vi "LDA_analogue_start_time_sync_PN.vi"(0 "Burst detect HW delay (s)":dbl=0.008, 4 "Correlation peak fit method":enum32{"Max", "Quadratic", "Gaussian"}(ring)=enum."Quadratic", 5 "Pulse high threshold (Volts)":dbl=2.5, 6 "Analogue dt (s)":dbl, 7 "Analogue LDA burst pulse array":dbl[](array[numeric]), 8 "LDA arrival Times":dbl[](array[numeric])) -> (1 "valid bursts checksum status":bool=TRUE, 2 "Absolute LDA times (s)":dbl[](array[numeric]), 3 "LDA start time rel. to Analogue (s)":dbl)   [LabVIEW 2011]
uses:
  <vilib>/Analysis/1siggen.llb/Ramp Pattern by Samples.vi
  <vilib>/Analysis/2dsp.llb/1D Cross Correlation (DBL).vi
  <vilib>/Analysis/polynomials.llb/Polynomial Roots (DBL).vi
  <vilib>/Analysis/polynomials.llb/nth Derivative of Polynomial (DBL).vi
  <vilib>/Analysis/NI_AALPro.lvlib
  <vilib>/Analysis/NI_AALBase.lvlib
panel:
  out "Xcorr LDA timings":cluster{"Ramp Pattern":dbl[], dbl[]}[](graph)
  in  "Pts. either side of peak to use in fit":i32=3
  out "Analogue LDA burst pulse array":cluster{"index (row)":dbl, dbl, "Vout":dbl[]}(graph)
  out "Thresholded LDA burst times (valid only)":cluster{"index (row)":dbl, dbl, "Vout":dbl[]}(graph)
  out "Thresholded LDA arr time checksum":i32
  out "Thresholded LDA burst times (valid + invalid)":cluster{"index (row)":dbl, dbl, "Vout":dbl[]}(graph)
  out "LDA counted pulses (valid + invalid)":i32
  out "LDA arr_t length":i32
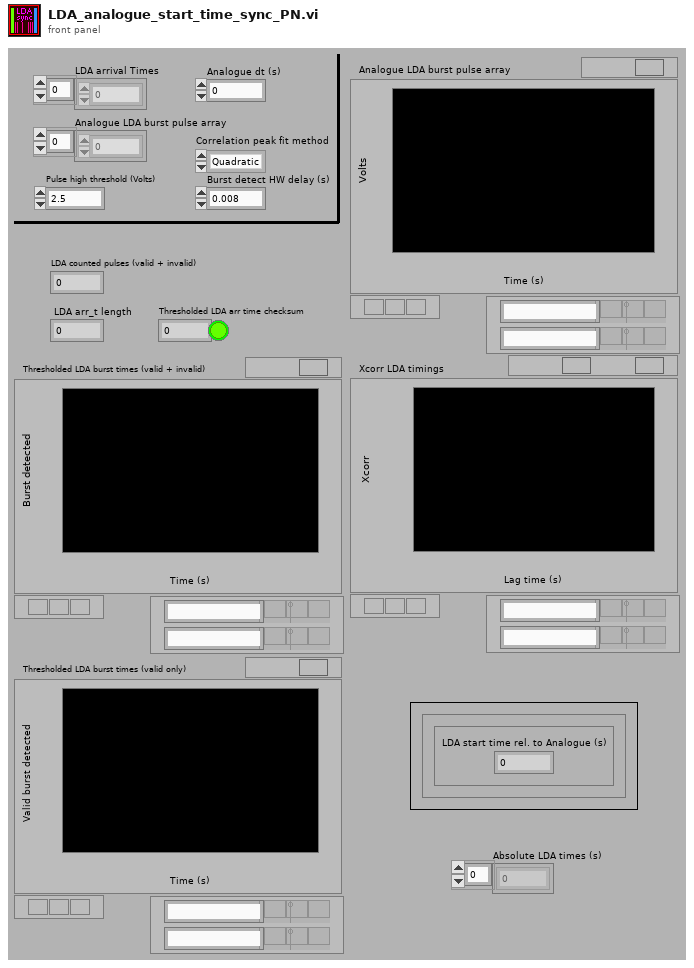
[diagram p1: front panel]
types:
  T1 = cluster{"index (row)":dbl, "Analogue dt (s)":dbl, "Vout":dbl[]}
  T2 = cluster{"index (row)":dbl, "Analogue dt (s)":dbl, "Analogue LDA burst pulse array":dbl[]}
  T3 = cluster{"Ramp Pattern":dbl[], "Best Gaussian Fit":dbl[]}[]
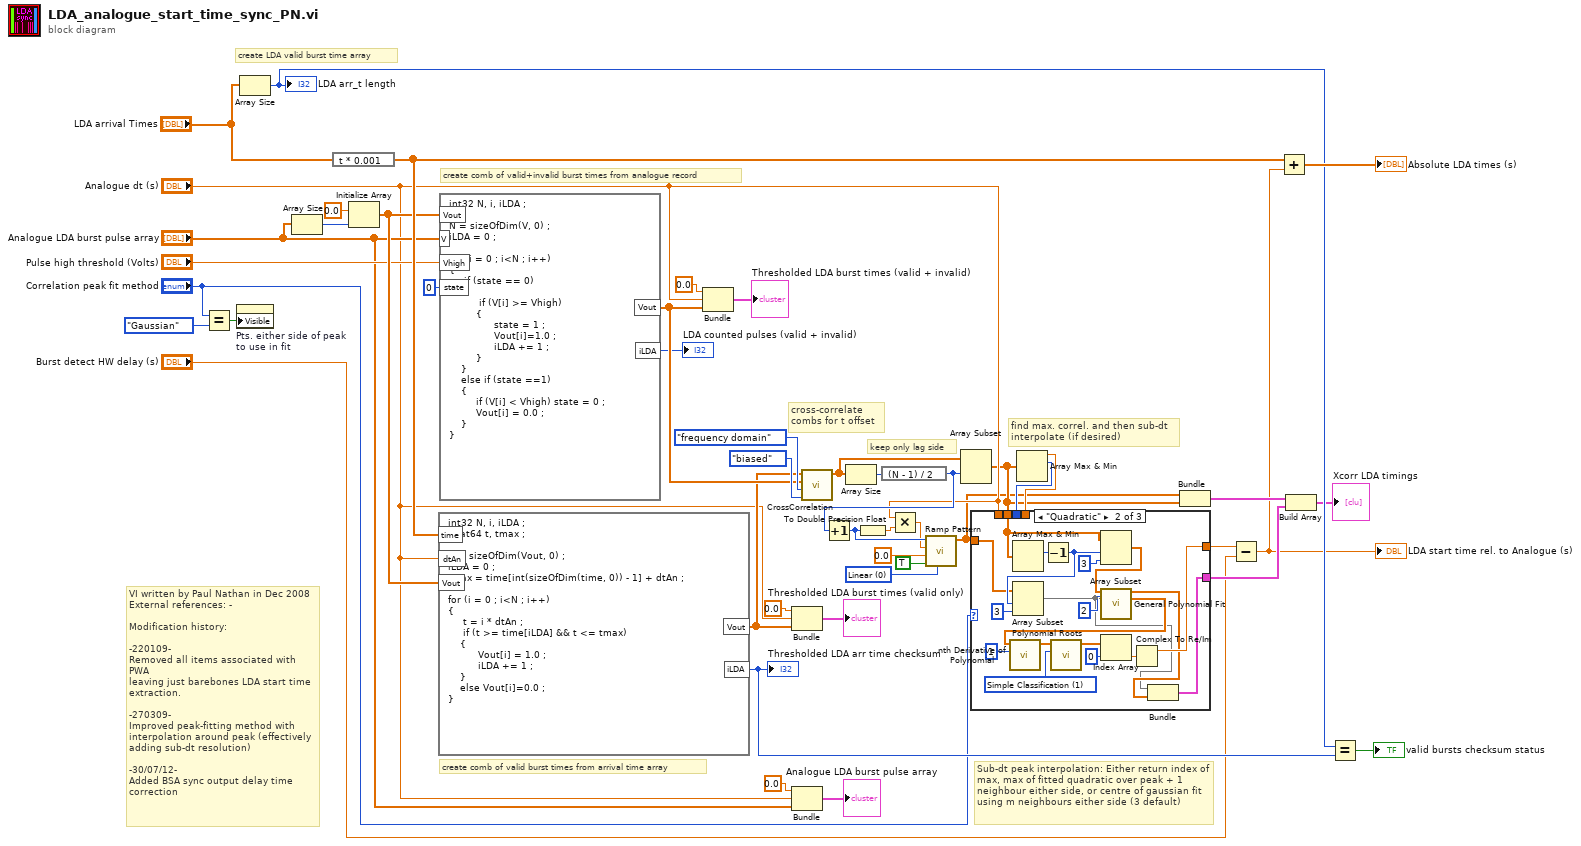
[diagram p0: block diagram]
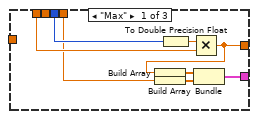
[diagram p2: hidden frame]
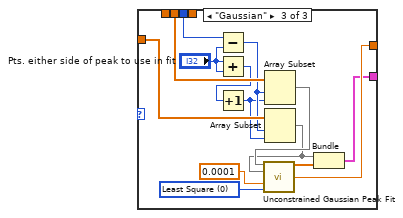
[diagram p3: hidden frame]
diagram:
  w13 = u16 0 items=["Linear", "Logarithmic"] ("type")
  # "find max. correl. and then sub-dt interpolate (if desired)"
  # "Sub-dt peak interpolation: Either return index of max, max of fitted quadratic over peak + 1 neighbour either side, or centre of gaussian fit using m neighbours either side (3 default)"
  # "create LDA valid burst time array"
  # "keep only lag side"
  # "cross-correlate combs for t offset"
  # "VI written by Paul Nathan in Dec 2008\nExternal references: -\n\nModification history:\n\n-220109-\nRemoved all items associated with PWA\nleaving just barebones LDA start time\nextraction.\n\n-270309-\nImproved peak-fitting method with interpolation around peak (effectively adding sub-dt resolution)\n\n-30/07/12-\nAdded BSA sync output delay time correction"
  # "create comb of valid+invalid burst times from analogue record"
  # "create comb of valid burst times from arrival time array"
  n1 = Equal?(x="Correlation peak fit method", y=enum32{"Max", "Quadratic", "Gaussian"}."Gaussian") -> (x = y?=w6:bool)
  n2 = property on="Pts. either side of peak to use in fit" class="DigNum (strict)"("Visible"=w6) -> ()  [unwired: 2 in, 2 out]
  n3 = Array Size(array="LDA arrival Times") -> (size(s)=w28:i32)
  "LDA arr_t length" <- w28
  n4 = Array Size(array="Analogue LDA burst pulse array") -> (size(s)=w33:i32)
  n5 = expression code="t * 0.001"("LDA arrival Times") -> (w34:dbl[])
  n6 = Initialize Array(0.0 ("element"), w33) -> (w32:dbl[])
  n7 = formula code="int32 N, i, iLDA ;\nfloat64 t, tmax ;\n\nN = sizeOfDim(Vout, 0) ;\niLDA = 0 ;\ntmax = time[int(sizeOfDim(time, 0)) - 1] + dtAn ;\n\nfor (i = 0 ; i<N ; i++)\n{\n     t = i * dtAn ;\n     if (t >= time[iLDA] && t <= tmax) \n    {\n          Vout[i] = 1.0 ;\n          iLDA += 1 ;\n    }\n    else Vout[i]=0.0 ;\n}"("dtAn"="Analogue dt (s)", "time"=w34, "Vout"=w32) -> ("Vout"=w37:dbl[], "iLDA"=w31:i32)
  "Thresholded LDA arr time checksum" <- w31
  n8 = formula code="int32 N, i, iLDA ;\n\nN = sizeOfDim(V, 0) ;\niLDA = 0 ;\n\nfor (i = 0 ; i<N ; i++)\n{\n     if (state == 0) \n    {\n          if (V[i] >= Vhigh)\n         {\n               state = 1 ;\n               Vout[i]=1.0 ;\n               iLDA += 1 ;\n         }\n    }\n    else if (state ==1)\n    {\n         if (V[i] < Vhigh) state = 0 ;\n         Vout[i] = 0.0 ;\n    }\n}"("V"="Analogue LDA burst pulse array", "Vhigh"="Pulse high threshold (Volts)", "state"=u8 0 ("input variable"), "Vout"=w32) -> ("Vout"=w38:dbl[], "iLDA"=→"LDA counted pulses (valid + invalid)":i32)
  n9 = Bundle("index (row)"=0.0, "Analogue dt (s)"="Analogue dt (s)", "Vout"=w38) -> (→"Thresholded LDA burst times (valid + invalid)":T1)  [unwired: 1 out]
  n10 = Bundle("index (row)"=0.0, "Analogue dt (s)"="Analogue dt (s)", "Vout"=w37) -> (→"Thresholded LDA burst times (valid only)":T1)  [unwired: 1 out]
  n11 = Bundle("index (row)"=0.0, "Analogue dt (s)"="Analogue dt (s)", "Analogue LDA burst pulse array"="Analogue LDA burst pulse array") -> (→"Analogue LDA burst pulse array":T2)  [unwired: 1 out]
  n12 = call-poly <vilib>:"CrossCorrelation.vi"("normalization"=enum32{"none", "unbiased", "biased"}."biased", "algorithm"=enum32{"direct", "frequency domain"}."frequency domain", "Y"=w38, "X"=w37) -> ("Rxy"=w35:dbl[])  [unwired: 7 out]
  n13 = Array Size(array=w35) -> (size(s)=w36:i32)
  n14 = expression code="(N - 1) / 2"(w36) -> (w15:i32)
  n15 = Increment(x=w15) -> (x+1=w22:i32)
  n16 = To Double Precision Float(number=w22) -> (double precision float=w20:dbl)
  n17 = Multiply(x="Analogue dt (s)", y=w20) -> (x*y=w21:dbl)
  n18 = call-poly <vilib>:"Ramp Pattern.vi"("type"=w13, "exclude end?"=TRUE, "start"=0.0, "end"=w21, "samples"=w22) -> ("Ramp Pattern"=w9:dbl[])  [unwired: 5 in, 1 out]
  n19 = Array Subset(array=w35, index=w15) -> (w10:dbl[])  [unwired: 1 in]
  n20 = Array Max & Min(array=w10) -> (max value=w11:dbl, max index (indices)=w12:i32)  [unwired: 2 out]
  n21 = case shown="\"Quadratic\"" "Correlation peak fit method" {
    tunnel: w10 -> [_ w62 w84]
    tunnel: [w47 w63 w86] -> w3
    tunnel: "Analogue dt (s)" -> [w54 _ _]
    tunnel: [w51 w60 w76] -> w8
    tunnel: w9 -> [_ w56 w81]
    tunnel: w12 -> [w52 _ w83]
    tunnel: w11 -> [w48 _ _]
    frame "Max" {
      n22 = Build Array(w48) -> (w50:dbl[])
      n23 = To Double Precision Float(number=w52) -> (double precision float=w53:dbl)
      n24 = Multiply(x=w53, y=w54) -> (x*y=w47:dbl)
      n25 = Build Array(w47) -> (w49:dbl[])
      n26 = Bundle(w49, w50) -> (w51:cluster{dbl[], dbl[]})  [unwired: 1 out]
    }
    frame "Quadratic" {
      w67 = u16 1 items=["General", "Simple Classification", "Refinement", "Advanced Refinement"] ("option")
      n27 = Array Max & Min(array=w62) -> (max index (indices)=w72:i32)  [unwired: 3 out]
      n28 = Decrement(x=w72) -> (x-1=w57:i32)
      n29 = Array Subset(array=w56, index=w57, length=3) -> (w55:dbl[])
      n30 = Array Subset(array=w62, index=w57, length=3) -> (w71:dbl[])
      n31 = call <vilib>:"General Polynomial Fit.vi"("Y"=w71, "polynomial order"=2, "X"=w55) -> ("Best Polynomial Fit"=w59:dbl[], "Polynomial Coefficients"=w61:dbl[])  [unwired: 9 in, 2 out]
      n32 = call-poly <vilib>:"nth Derivative of Polynomial.vi"("order"=1, "P(x)"=w61) -> ("Nth Derivative of P(x)"=w68:dbl[])  [unwired: 9 out]
      n33 = call-poly <vilib>:"Polynomial Roots.vi"("option"=w67, "P(x)"=w68) -> ("Roots"=w66:cdb[])  [unwired: 9 out]
      n34 = Index Array(array=w66, index=0) -> (element=w64:cdb)
      n35 = Complex To Re/Im(x + iy=w64) -> (x=w63:dbl)  [unwired: 1 out]
      n36 = Bundle(w55, "Best Polynomial Fit"=w59) -> (w60:cluster{dbl[], "Best Polynomial Fit":dbl[]})  [unwired: 1 out]
    }
    frame "Gaussian" {
      w85 = u16 0 items=["Least Square", "Least Absolute Residual", "Bisquare"] ("method")
      n37 = Subtract(x=w83, y="Pts. either side of peak to use in fit") -> (x-y=w80:i32)
      n38 = Add(x="Pts. either side of peak to use in fit", y="Pts. either side of peak to use in fit") -> (x+y=w74:i32)
      n39 = Increment(x=w74) -> (x+1=w75:i32)
      n40 = Array Subset(array=w84, index=w80, length=w75) -> (w79:dbl[])
      n41 = Array Subset(array=w81, index=w80, length=w75) -> (w77:dbl[])
      n42 = call <vilib>:"Unconstrained Gaussian Peak Fit.vi"("Y"=w79, "X"=w77, "tolerance"=0.0001, "method"=w85) -> ("Best Gaussian Fit"=w78:dbl[], "center"=w86:dbl)  [unwired: 6 in, 4 out]
      n43 = Bundle(w77, "Best Gaussian Fit"=w78) -> (w76:cluster{dbl[], "Best Gaussian Fit":dbl[]})  [unwired: 1 out]
    }
  }
  n44 = Bundle("Ramp Pattern"=w9, w10) -> (w16:cluster{"Ramp Pattern":dbl[], dbl[]})  [unwired: 1 out]
  n45 = Subtract(x=w3, y="Burst detect HW delay (s)") -> (x-y=w2:dbl)
  "LDA start time rel. to Analogue (s)" <- w2
  n46 = Add(x=w34, y=w2) -> (x+y=→"Absolute LDA times (s)":dbl[])
  n47 = Build Array(w16, w8) -> (→"Xcorr LDA timings":T3)
  n48 = Equal?(x=w28, y=w31) -> (x = y?=→"valid bursts checksum status":bool)
